vi "L1_subset.vi"(2 "subset length":i32(slide)=307 scale=0.0..800.0, 3 "in array":dbl[](array[numeric])) -> (0 "Index":i32, 1 "subarray":dbl[](array[numeric]))   [LabVIEW 2009]
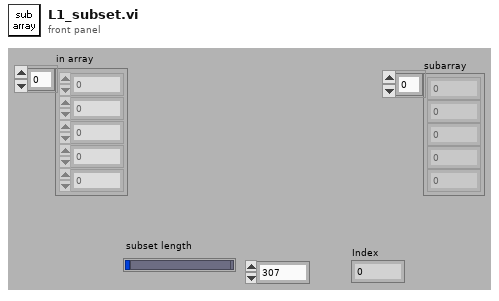
[diagram p1: front panel]
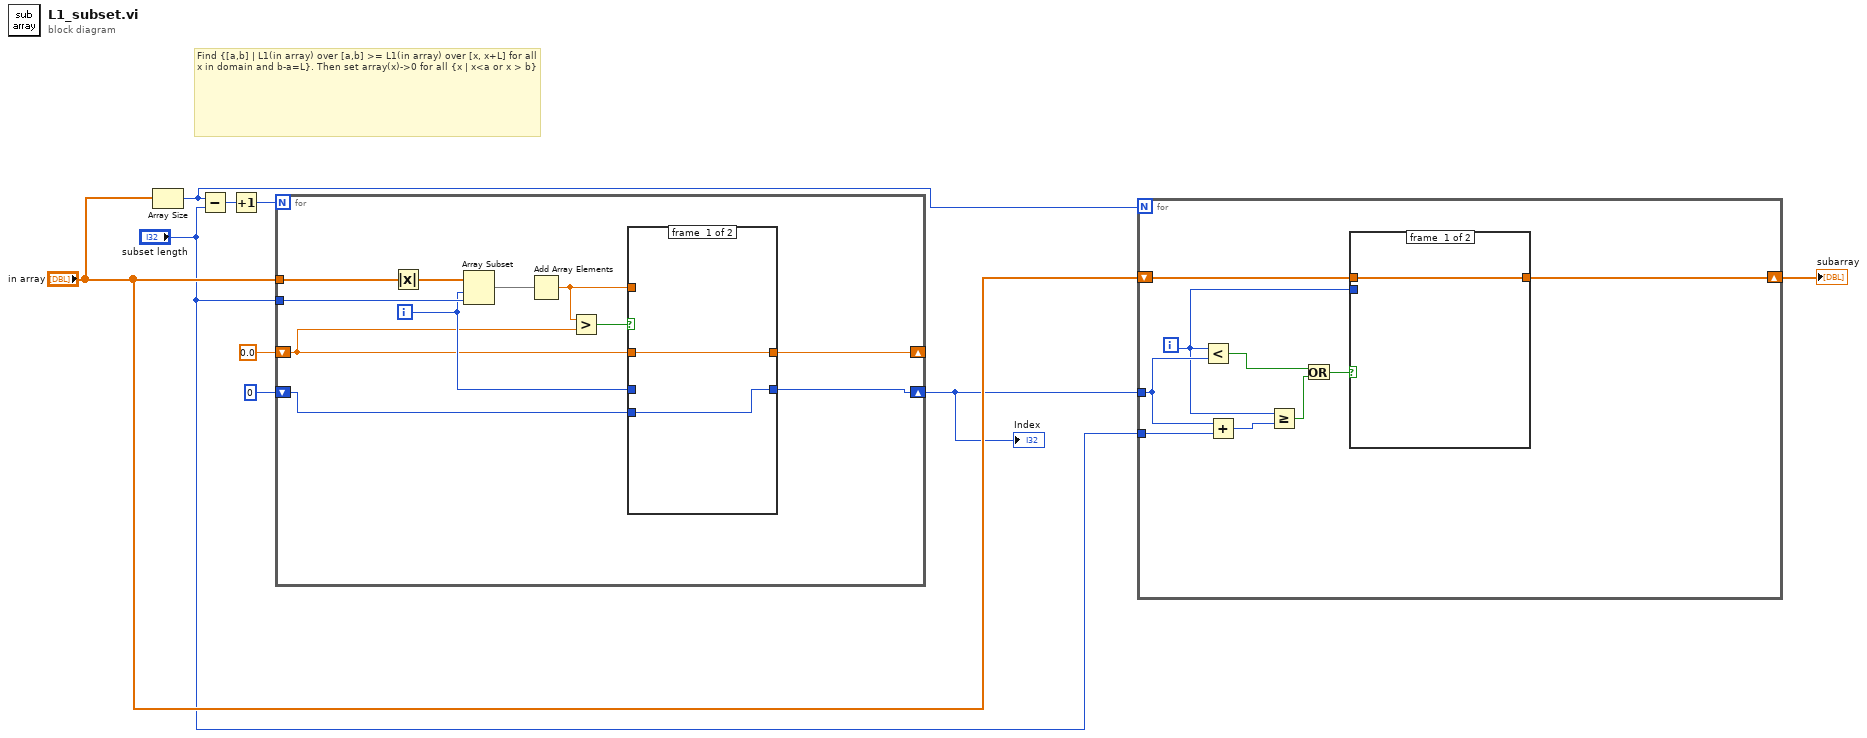
[diagram p0: block diagram]
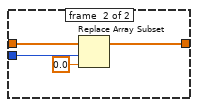
[diagram p2: hidden frame]
diagram:
  # "Find {[a,b] | L1(in array) over [a,b] >= L1(in array) over [x, x+L] for all x in domain and b-a=L}. Then set array(x)->0 for all {x | x<a or x > b}"
  n1 = Array Size(array="in array") -> (size(s)=w1:i32)
  n2 = Subtract(x=w1, y="subset length") -> (x-y=w9:i32)
  n3 = Increment(x=w9) -> (x+1=w8:i32)
  n4 = for {
    N: w8 -> [_]
    tunnel: "in array" -> [w20]
    tunnel: "subset length" -> [w18]
    shift-right: [w14] -> _
    shift-left: 0.0 -> [w10]
    shift-right: [w13] -> w4
    shift-left: 0 -> [w11]
    i -> [w12]
    n5 = Absolute Value(x=w20) -> (abs(x)=w19:dbl[])
    n6 = Array Subset(array=w19, index=w12, length=w18) -> (w17:dbl[])
    n7 = Add Array Elements(numeric array=w17) -> (sum=w15:dbl)
    n8 = Greater?(x=w15, y=w10) -> (0:w16:bool)
    n9 = case shown="True" w16 {
      tunnel: w15 -> [_ w24]
      tunnel: [w21 w24] -> w14
      tunnel: [w22 w23] -> w13
      tunnel: w12 -> [_ w23]
      tunnel: w11 -> [w22 _]
      tunnel: w10 -> [w21 _]
      frame #0 {
      }
      frame #1 {
      }
    }
  }
  "Index" <- w4
  n10 = for {
    N: w1 -> [_]
    tunnel: w4 -> [w32]
    shift-right: [w25] -> w2
    shift-left: "in array" -> [w28]
    tunnel: "subset length" -> [w31]
    i -> [w26]
    n11 = Less?(x=w26, y=w32) -> (x < y?=w33:bool)
    n12 = Add(x=w32, y=w31) -> (x+y=w30:i32)
    n13 = Greater Or Equal?(x=w26, y=w30) -> (x >= y?=w29:bool)
    n14 = Or(x=w33, y=w29) -> (x .or. y?=w27:bool)
    n15 = case shown="False" w27 {
      tunnel: w28 -> [w34 w38]
      tunnel: w26 -> [_ w36]
      tunnel: [w34 w35] -> w25
      frame #0 {
      }
      frame #1 {
        n16 = Replace Array Subset(array=w38, new element=0.0 ("new element/subarray"), index=w36) -> (w35:dbl[])
      }
    }
  }
  "subarray" <- w2
